vi "MGI Statistical Histogram.vi"(0 "X[]":dbl[](array[numeric]) format="%.2f") -> (1 "Mean":dbl format="%.2f", 2 "Standard Deviation":dbl format="%.2f", 3 "Histogram":cluster{dbl, "standard deviation":dbl, i32[]}(graph))   [LabVIEW 2020]
doc: "Create a histogram based on +/-3 standard deviations and outliers.\n\nAuthored by David A Moore\nsupport@mooregoodideas.com\nwww.mooregoodideas.com\n\nCopyright (c) 2010, Moore Good Ideas, Inc.\n\nAll rights reserved.\n\nRedistribution and use in source and binary forms, with or without modification, are permitted provided that the following conditions are met:\n\n * Redistributions of source code must retain the above copyright notice, this list of conditions and the following disclaimer.\n * Redistributions in binary form must reproduce the above copyright notice, this list of conditions and the following disclaimer in the documentation and/or other materials provided with the distribution.\n * Neither the name of Moore Good Ideas, Inc. nor the names of its contributors may be used to endorse or promote products derived from this software without specific prior written permission.\n\nTHIS SOFTWARE IS PROVIDED BY THE COPYRIGHT HOLDERS AND CONTRIBUTORS \"AS IS\" AND ANY EXPRESS OR IMPLIED WARRANTIES, INCLUDING, BUT NOT LIMITED TO, THE IMPLIED WARRANTIES OF MERCHANTABILITY AND FITNESS FOR A PARTICULAR PURPOSE ARE DISCLAIMED. IN NO EVENT SHALL THE COPYRIGHT OWNER OR CONTRIBUTORS BE LIABLE FOR ANY DIRECT, INDIRECT, INCIDENTAL, SPECIAL, EXEMPLARY, OR CONSEQUENTIAL DAMAGES (INCLUDING, BUT NOT LIMITED TO, PROCUREMENT OF SUBSTITUTE GOODS OR SERVICES; LOSS OF USE, DATA, OR PROFITS; OR BUSINESS INTERRUPTION) HOWEVER CAUSED AND ON ANY THEORY OF LIABILITY, WHETHER IN CONTRACT, STRICT LIABILITY, OR TORT (INCLUDING NEGLIGENCE OR OTHERWISE) ARISING IN ANY WAY OUT OF THE USE OF THIS SOFTWARE, EVEN IF ADVISED OF THE POSSIBILITY OF SUCH DAMAGE."
uses:
  <vilib>/Analysis/NI_AALBase.lvlib
  <vilib>/Analysis/NI_AALPro.lvlib
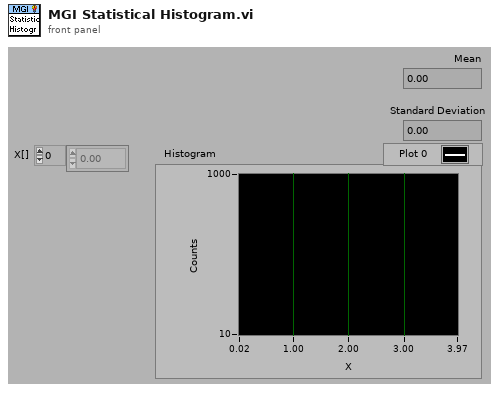
[diagram p1: front panel]
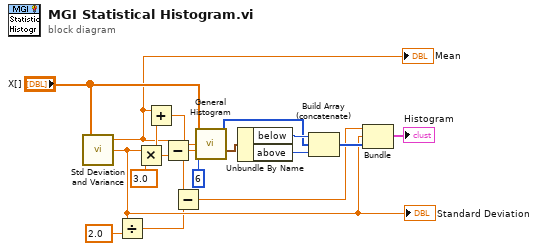
[diagram p0: block diagram]
diagram:
  n1 = call <vilib>:"Std Deviation and Variance.vi"("X"="X[]") -> ("mean"=w14:dbl, "standard deviation"=w3:dbl)  [unwired: 1 in, 1 out]
  "Mean" <- w14
  "Standard Deviation" <- w3
  n2 = Divide(x=w3, y=2.0) -> (x/y=w1:dbl)
  n3 = Multiply(x=w3, y=3.0) -> (x*y=w15:dbl)
  n4 = Add(x=w14, y=w15) -> (x+y=w13:dbl)
  n5 = Subtract(x=w14, y=w15) -> (x-y=w6:dbl)
  n6 = Subtract(x=w6, y=w1) -> (x-y=w5:dbl)
  n7 = call <vilib>:"General Histogram.vi"("X"="X[]", "max"=w13, "min"=w6, "# bins"=6) -> ("Histogram"=w8:i32[], "# outside"=w11:cluster{"total":i32, "below":i32, "above":i32})  [unwired: 7 in, 3 out]
  n8 = Unbundle By Name(w11) -> ("below"=w10:i32, "above"=w9:i32)
  n9 = Build Array (concatenate)(w10, w8, w9) -> (w7:i32[])
  n10 = Bundle(w5, "standard deviation"=w3, w7) -> (→"Histogram":cluster{dbl, "standard deviation":dbl, i32[]})  [unwired: 1 in]
